vi "CRYSet Messages Front Panel.vi"(11 "Vi Ref":refnum<vi>) -> ()   [LabVIEW 2013]
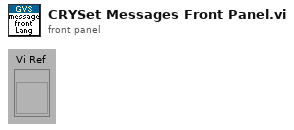
[diagram p1: front panel]
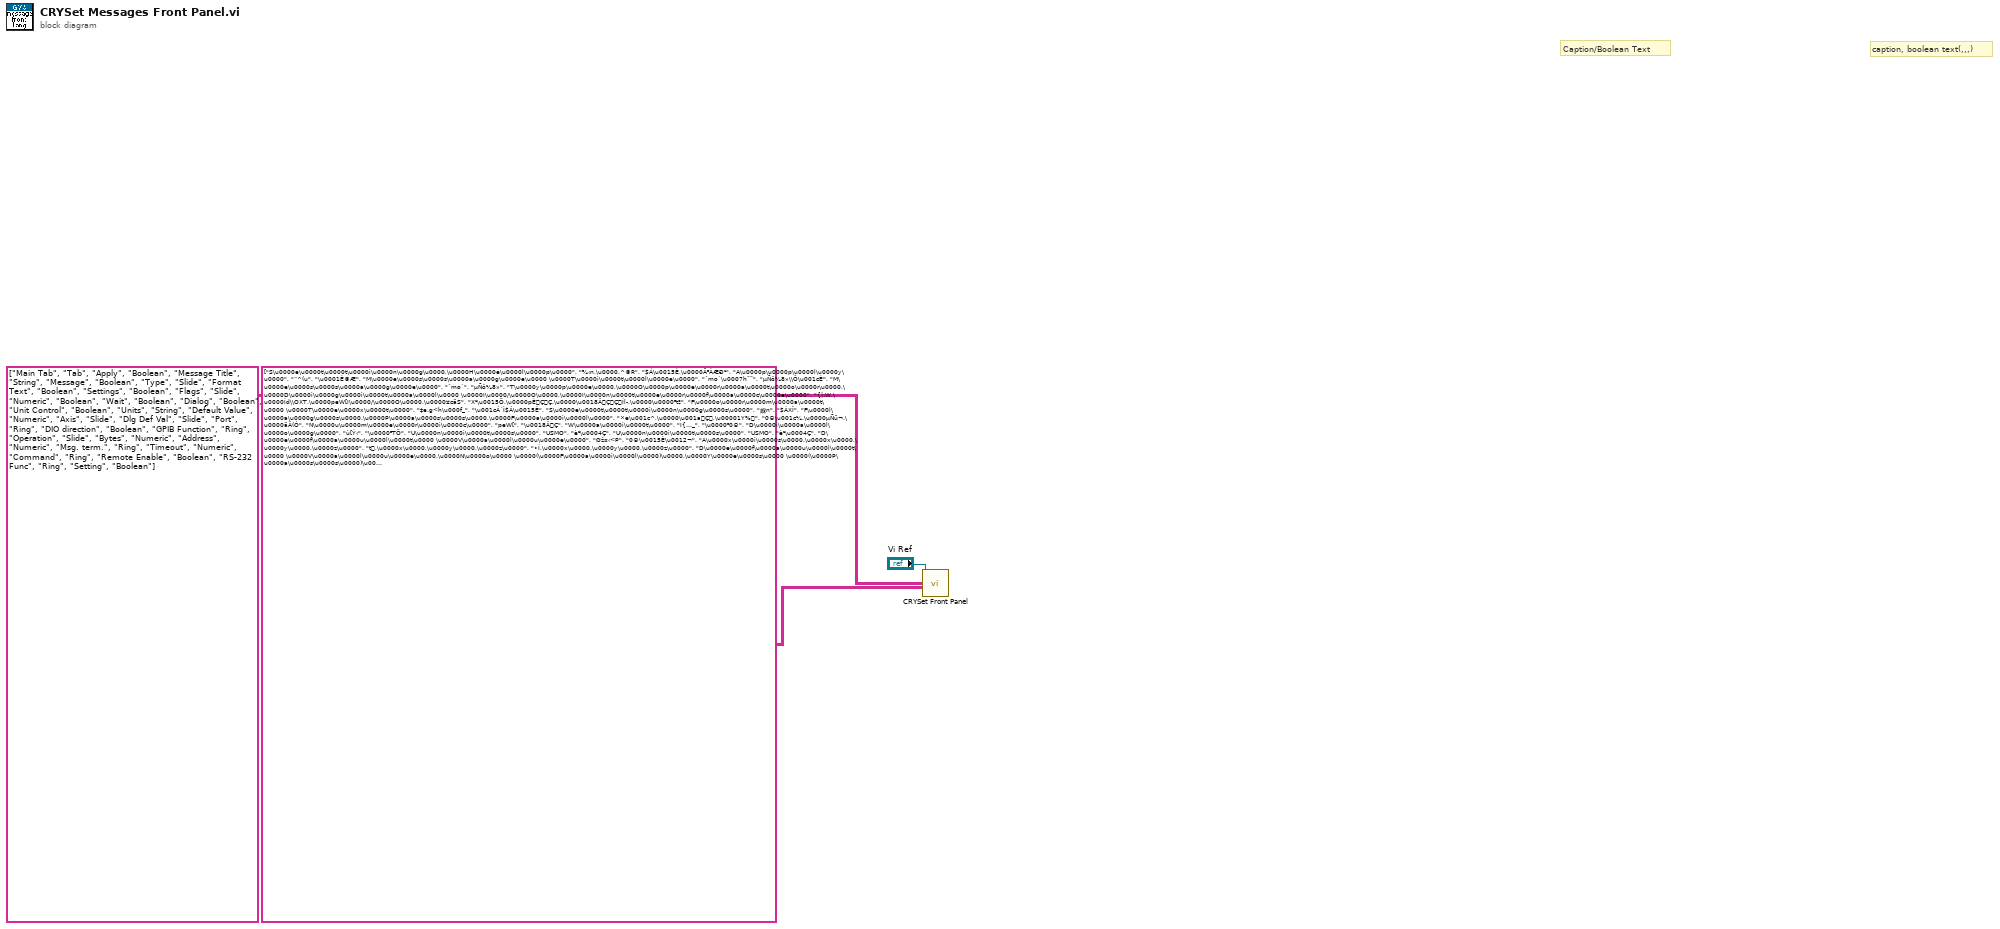
[diagram p0: block diagram]
diagram:
  # "Caption, Tab Page, Multilist Header, Button 4"
  # "Control Type"
  # "Control Name and Tab"
  # "caption, boolean text(,,,)"
  # "Caption/Boolean Text"
  n1 = call "CRYSet Front Panel.vi"("Caption(Boolean Text)"=string[][] [["S\u0000e\u0000t\u0000t\u0000i\u0000n\u0000g\u0000,\u0000H\u0000e\u0000l\u0000p\u0000", "¾‹n,\u0000.^©R", "$Á\u0015È,\u0000Ä³ÀÆÐ¹"], ["A\u0000p\u0000p\u0000l\u0000y\u0000", "”^(u", "\u0001È©Æ"], ["M\u0000e\u0000s\u0000s\u0000a\u0000g\u0000e\u0000 \u0000T\u0000i\u0000t\u0000l\u0000e\u0000", "ˆmo`\u0007h˜˜", "µÑô¼8»\\Ô\u001cÈ"], ["M\u0000e\u0000s\u0000s\u0000a\u0000g\u0000e\u0000", "ˆmo`", "µÑô¼8»"], ["T\u0000y\u0000p\u0000e\u0000,\u0000O\u0000p\u0000e\u0000r\u0000a\u0000t\u0000o\u0000r\u0000,\u0000D\u0000i\u0000g\u0000i\u0000t\u0000a\u0000l\u0000 \u0000I\u0000/\u0000O\u0000,\u0000I\u0000n\u0000t\u0000e\u0000r\u0000f\u0000a\u0000c\u0000e\u0000", "{|‹W,\u0000Íd\\OXT,\u0000peW[I\u0000/\u0000O\u0000,\u0000¥cãS", "X¹\u0015Ö,\u0000pÈÇÇ,\u0000\u0018ÂÇÇÍl­,\u0000\u0000³tº"], ["F\u0000o\u0000r\u0000m\u0000a\u0000t\u0000 \u0000T\u0000e\u0000x\u0000t\u0000", "‡e,g<h\u000f_", "\u001cÁ´Ì$Á\u0015È"], ["S\u0000e\u0000t\u0000t\u0000i\u0000n\u0000g\u0000s\u0000", "緥n", "$ÁXÎ"], ["F\u0000l\u0000a\u0000g\u0000s\u0000,\u0000P\u0000a\u0000s\u0000s\u0000,\u0000F\u0000a\u0000i\u0000l\u0000", "×e\u001c^,\u0000\u001aÇ,\u00001Y%", "0®\u001c¼,\u0000µÑü¬,\u0000äÂ(Ó"], ["N\u0000u\u0000m\u0000e\u0000r\u0000i\u0000c\u0000", "peW[", "\u0018ÂÇ"], ["W\u0000a\u0000i\u0000t\u0000", "I{…_", "\u0000³0®"], ["D\u0000i\u0000a\u0000l\u0000o\u0000g\u0000", "ù[Ý‹", "\u0000³TÖ"], ["U\u0000n\u0000i\u0000t\u0000s\u0000", "USMO", "è²\u0004Ç"], ["U\u0000n\u0000i\u0000t\u0000s\u0000", "USMO", "è²\u0004Ç"], ["D\u0000e\u0000f\u0000a\u0000u\u0000l\u0000t\u0000 \u0000V\u0000a\u0000l\u0000u\u0000e\u0000", "Øž¤‹<P", "0®\u0015È\u0012¬"], ["A\u0000x\u0000i\u0000s\u0000,\u0000x\u0000,\u0000y\u0000,\u0000z\u0000", "t,\u0000x\u0000,\u0000y\u0000,\u0000z\u0000", "•Í,\u0000x\u0000,\u0000y\u0000,\u0000z\u0000"], ["D\u0000e\u0000f\u0000a\u0000u\u0000l\u0000t\u0000 \u0000V\u0000a\u0000l\u0000u\u0000e\u0000,\u0000N\u0000o\u0000 \u0000(\u0000F\u0000a\u0000i\u0000l\u0000)\u0000,\u0000Y\u0000e\u0000s\u0000 \u0000(\u0000P\u0000a\u0000s\u0000s\u0000)\u0000", "Ø¤<P,\u0000&T \u0000(\u00001Y%)\u0000,\u0000/f \u0000(\u0000\u001aÇ)\u0000", "0®\u0015È\u0012¬,\u0000DÅÈ² \u0000(\u0000äÂ(Ó)\u0000,\u0000\bÆ \u0000(\u0000µÑü¬)\u0000"], ["P\u0000o\u0000r\u0000t\u0000", "ïzãS", "ìÓl­"], ["O\u0000u\u0000t\u0000p\u0000u\u0000t\u0000,\u0000I\u0000n\u0000p\u0000u\u0000t\u0000", "úQ,\u0000eQ", "œÍl­,\u0000…Çl­"], ["F\u0000u\u0000n\u0000c\u0000t\u0000i\u0000o\u0000n\u0000", "ŸRý€", "0®¥²"], ["O\u0000p\u0000e\u0000r\u0000a\u0000t\u0000i\u0000o\u0000n\u0000,\u0000R\u0000e\u0000a\u0000d\u0000,\u0000W\u0000r\u0000i\u0000t\u0000e\u0000", "Íd\\O,\u0000û‹,\u0000™Q", "pÈ‘Ç,\u0000}Ç0®,\u0000ðÄ0®"], ["b\u0000y\u0000t\u0000e\u0000s\u0000", "MOpe", "\u0014¼tÇ¸Ò\u0018Â"], ["A\u0000d\u0000d\u0000r\u0000e\u0000s\u0000s\u0000", "0W@W", "üÈŒÁ"], ["M\u0000s\u0000g\u0000.\u0000 \u0000t\u0000e\u0000r\u0000m\u0000.\u0000", "y˜îv", "mÕ©º"], ["T\u0000i\u0000m\u0000e\u0000o\u0000u\u0000t\u0000", "‚f\\P", "¼¹ÜÂ\u0015ÈÀÉ"], ["C\u0000o\u0000m\u0000m\u0000a\u0000n\u0000d\u0000", "}TäN", "…º9¸"], ["R\u0000e\u0000m\u0000o\u0000t\u0000e\u0000 \u0000E\u0000n\u0000a\u0000b\u0000l\u0000e\u0000", "܏\u000bz/T(u", "ÐÆ©¬\u0000¬¥²"], ["F\u0000u\u0000n\u0000c\u0000t\u0000i\u0000o\u0000n\u0000", "ŸRý€", "0®¥²"], ["S\u0000e\u0000t\u0000t\u0000i\u0000n\u0000g\u0000", "緥n", "$Á\u0015È"]], "Control ID and Type(Label Name, Type)"=string[][] [["Main Tab", "Tab"], ["Apply", "Boolean"], ["Message Title", "String"], ["Message", "Boolean"], ["Type", "Slide"], ["Format Text", "Boolean"], ["Settings", "Boolean"], ["Flags", "Slide"], ["Numeric", "Boolean"], ["Wait", "Boolean"], ["Dialog", "Boolean"], ["Unit Control", "Boolean"], ["Units", "String"], ["Default Value", "Numeric"], ["Axis", "Slide"], ["Dlg Def Val", "Slide"], ["Port", "Ring"], ["DIO direction", "Boolean"], ["GPIB Function", "Ring"], ["Operation", "Slide"], ["Bytes", "Numeric"], ["Address", "Numeric"], ["Msg. term.", "Ring"], ["Timeout", "Numeric"], ["Command", "Ring"], ["Remote Enable", "Boolean"], ["RS-232 Func", "Ring"], ["Setting", "Boolean"]], "Vi Ref"="Vi Ref") -> ()  [unwired: 9 in]
